vi "Add Edge.vi"(11 "Abstract Graph in":refnum<class "Abstract Graph.lvclass">) -> (3 "Abstract Graph out":refnum<class "Abstract Graph.lvclass">)   [LabVIEW 2021, in "GraphLib.lvlib" / "Abstract Graph.lvclass"]
uses:
  Abstract Graph.lvclass
  Cluster - Edge.ctl
  Abstract Graph.lvclass/Abstract Graph.ctl
  GraphLib.lvlib
panel:
  in  "Edge":T1={"Node A"=variant(cluster{"Value":variant, "Child Node IDs":string[], "Attributes":map{string, string}} {"Value"=variant, "Child Node IDs"=[], "Attributes"={}}), "Node B"=variant(cluster{"Value":variant, "Child Node IDs":string[], "Attributes":map{string, string}} {"Value"=variant, "Child Node IDs"=[], "Attributes"={}}), "Attributes"={}}
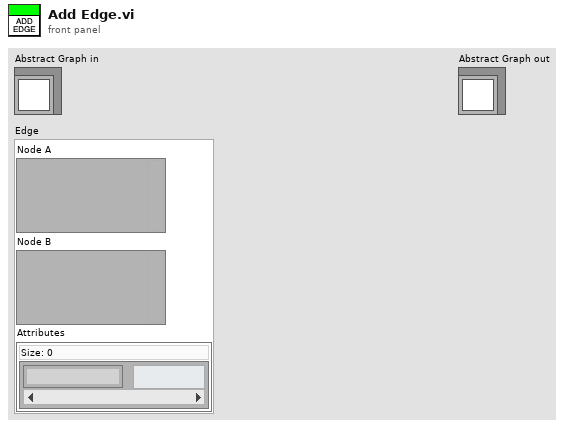
[diagram p1: front panel]
types:
  T1 = typedef "GraphLib.lvlib/Cluster - Edge.ctl" = cluster{"Node A":variant, "Node B":variant, "Attributes":map{string, string}}
  T2 = typedef "GraphLib.lvlib/Cluster - Graph Node.ctl" = cluster{"Value":variant, "Child Node IDs":set{string}, "Attributes":map{string, string}}
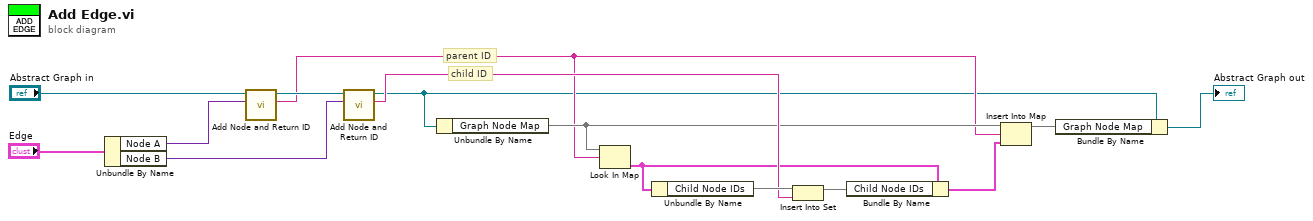
[diagram p0: block diagram]
diagram:
  # "child ID"
  # "parent ID"
  n1 = Unbundle By Name("Edge") -> ("Node A"=w13:variant, "Node B"=w11:variant)
  n2 = call-dynamic "Add Node and Return ID.vi"("Node"=w13, "Abstract Graph in"="Abstract Graph in") -> ("Node ID"=w4:string, "Abstract Graph out"=w12:refnum<class "Abstract Graph.lvclass">)  [unwired: 7 in, 1 out]
  n3 = call-dynamic "Add Node and Return ID.vi"("Node"=w11, "Abstract Graph in"=w12) -> ("Node ID"=w9:string, "Abstract Graph out"=w3:refnum<class "Abstract Graph.lvclass">)  [unwired: 7 in, 1 out]
  n4 = Unbundle By Name(w3) -> ("Graph Node Map"=w6:map{string, T2})
  n5 = Look In Map(map=w6, key=w4) -> (value=w8:T2)  [unwired: 1 in, 1 out]
  n6 = Unbundle By Name(w8) -> ("Child Node IDs"=w10:set{string})
  n7 = Insert Into Set(10:w9, 11:w10) -> (3:w7:set{string})  [unwired: 1 out]
  n8 = Bundle By Name(cluster=w8, "Child Node IDs"=w7) -> (w5:T2)
  n9 = Insert Into Map(map in=w6, key=w4, value=w5) -> (map out=w2:map{string, T2})  [unwired: 2 out]
  n10 = Bundle By Name(cluster=w3, "Graph Node Map"=w2) -> (→"Abstract Graph out":refnum<class "Abstract Graph.lvclass">)
